vi "Close Module If Already Open.vi"(8 "error in (no error)":errorcluster, 10 "Menu Type":enum16{"Root", "Sub", "Child"}(ring), 11 "Module List":string[](array[string])) -> (0 "error out":errorcluster)   [LabVIEW 2019, in "Menu Module.lvlib"]
uses:
  Menu Module.lvlib
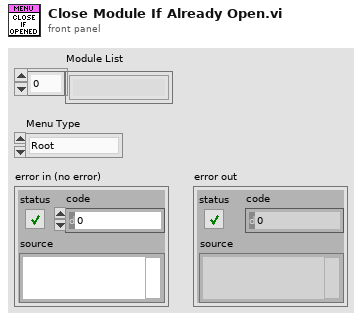
[diagram p1: front panel]
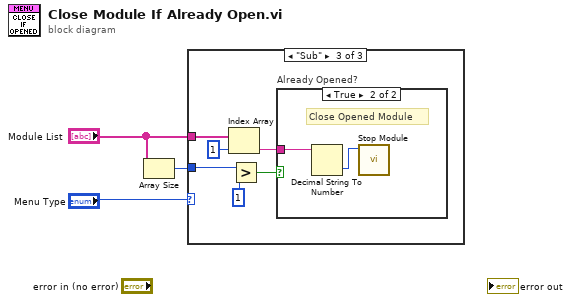
[diagram p0: block diagram]
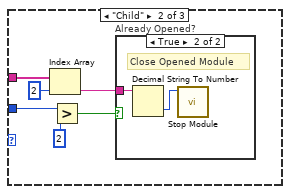
[diagram p3: hidden frame]
diagram:
  n1 = Array Size(array="Module List") -> (size(s)=w2:i32)
  n2 = case shown="\"Sub\"" "Menu Type" {
    tunnel: w2 -> [_ w9 w17]
    tunnel: "Module List" -> [_ w6 w14]
    frame "Root", Default {
    }
    frame "Child" {
      n3 = Index Array(array=w6, index=2) -> (element=w4:string)
      n4 = Greater?(x=w9, y=2) -> (0:w7:bool)
      n5 = case "Already Opened?" shown="True" w7 {
        tunnel: w4 -> [_ w10]
        frame False {
        }
        frame True {
          # "Close Opened Module"
          n6 = Decimal String To Number(string=w10) -> (number=w11:i32)  [unwired: 2 in, 1 out]
          n7 = call "Stop Module.vi"("Module ID"=w11) -> ()  [unwired: 10 in, 1 out]
        }
      }
    }
    frame "Sub" {
      n8 = Index Array(array=w14, index=1) -> (element=w12:string)
      n9 = Greater?(x=w17, y=1) -> (0:w15:bool)
      n10 = case "Already Opened?" shown="True" w15 {
        tunnel: w12 -> [_ w18]
        frame False {
        }
        frame True {
          # "Close Opened Module"
          n11 = Decimal String To Number(string=w18) -> (number=w19:i32)  [unwired: 2 in, 1 out]
          n12 = call "Stop Module.vi"("Module ID"=w19) -> ()  [unwired: 10 in, 1 out]
        }
      }
    }
  }
